vi "User32dllAPI.FrontMostWindow.vi"(8 "error in (no error)":errorcluster, 11 "hWnd":i32) -> (0 "error out":errorcluster, 3 "hWnd out":i32)   [LabVIEW 2019, in "Tools.lvlib"]
uses:
  Tools.lvlib
  user32.dll
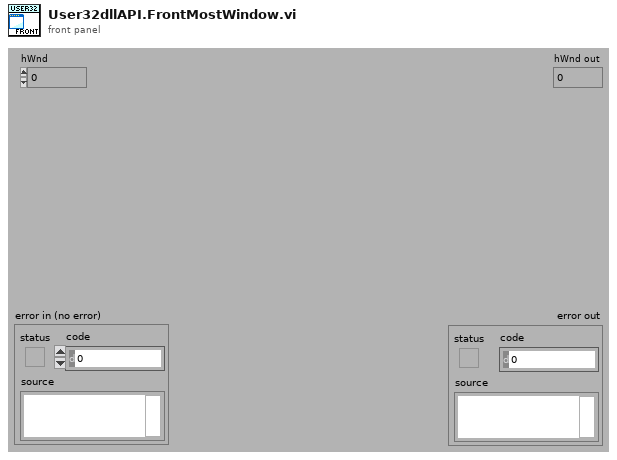
[diagram p1: front panel]
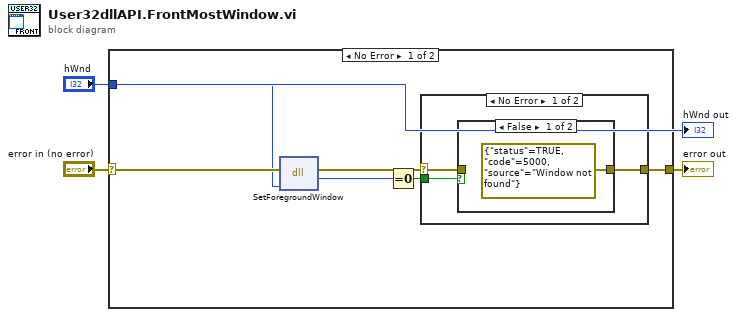
[diagram p0: block diagram]
diagram:
  n1 = case shown="No Error" "error in (no error)" {
    selector: "error in (no error)" -> [w7 w16]
    tunnel: [w8 w16] -> w2
    tunnel: "hWnd" -> [w4 _]
    frame No Error {
      n2 = dll-call lib="USER32.DLL" fn="SetForegroundWindow"(error in=w7, "hWnd"=w4) -> (error out=w6:errorcluster, "result"=w5:i32)  [unwired: 3 in, 1 out]
      n3 = Equal To 0?(x=w5) -> (x = 0?=w9:bool)
      n4 = case shown="No Error" w6 {
        selector: w6 -> [w10 w15]
        tunnel: w9 -> [w12 _]
        tunnel: [w11 w15] -> w8
        frame No Error {
          n5 = case shown="False" w12 {
            tunnel: [errorcluster {"status"=TRUE, "code"=5000, "source"="Window not found"} ("error out") w14] -> w11
            tunnel: w10 -> [_ w14]
            frame False {
            }
            frame True {
            }
          }
        }
        frame Error {
        }
      }
    }
    frame Error {
    }
  }
  "error out" <- w2
  "hWnd out" <- "hWnd"
